vi "Auto Scroll Tree.vi"(8 "error in":errorcluster, 10 "TreeControl in":refnum<vi>, 11 "Recent Root Tags Map":refnum<vi>) -> (0 "error out":errorcluster)   [LabVIEW 2025, in "CAN-LIN Raw Bus Capture UI.lvlib"]
doc: "This VI creates a buffer, and checks if the buffer size is more then 19, then it deletes the oldest element, adds the new one to the end, and sets the TREE's top left cell to the oldest one. So the latest 20 element will be shown in the tree."
uses:
  CAN-LIN Raw Bus Capture UI.lvlib
  <vilib>/Utility/miscctls.llb/LVNodeAndColumnTypeDef.ctl
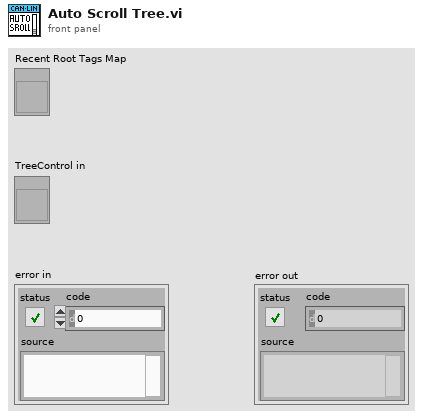
[diagram p1: front panel]
types:
  T1 = typedef "LVNodeAndColumnTypeDef.ctl" = cluster{"Node":string, "Column":i32}
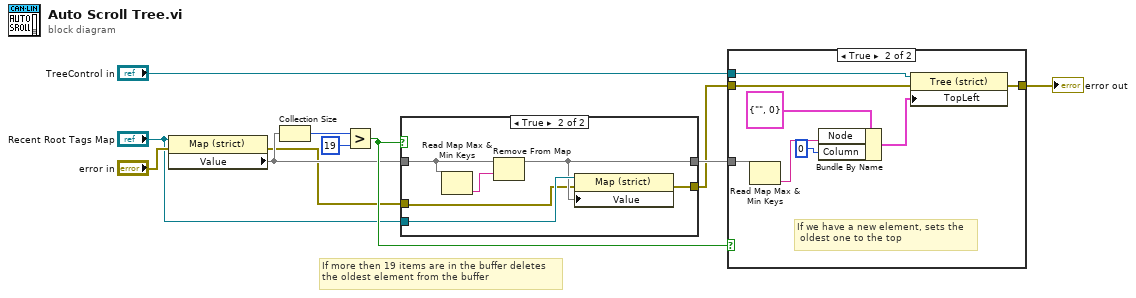
[diagram p0: block diagram]
diagram:
  # "If more then 19 items are in the buffer deletes\nthe oldest element from the buffer"
  n1 = property class="Map (strict)"(reference="Recent Root Tags Map", error in="error in") -> (error out=w2:errorcluster, "Value"=w6:map{string, string})  [unwired: 1 out]
  n2 = Collection Size(1:w6) -> (0:w7:i32)
  n3 = Greater?(x=w7, y=19) -> (0:w9:bool)
  n4 = case shown="True" w9 {
    tunnel: w6 -> [w13 w19]
    tunnel: [w13 w16] -> w5
    tunnel: "Recent Root Tags Map" -> [_ w17]
    tunnel: w2 -> [w12 w15]
    tunnel: [w12 w14] -> w1
    frame False {
    }
    frame True {
      n5 = Read Map Max & Min Keys(11:w19) -> (1:w18:string)  [unwired: 1 out]
      n6 = Remove From Map(10:w18, 11:w19) -> (3:w16:map{string, string})  [unwired: 2 out]
      n7 = property class="Map (strict)"(reference=w17, error in=w15, "Value"=w16) -> (error out=w14:errorcluster)  [unwired: 1 out]
    }
  }
  n8 = case shown="True" w9 {
    tunnel: [w20 w28] -> w11
    tunnel: "TreeControl in" -> [_ w27]
    tunnel: w1 -> [w20 w26]
    tunnel: w5 -> [_ w22]
    frame False {
    }
    frame True {
      # "If we have a new element, sets the\n oldest one to the top"
      n9 = Read Map Max & Min Keys(11:w22) -> (1:w21:string)  [unwired: 1 out]
      n10 = Bundle By Name(cluster=T1 {"Node"="", "Column"=0} ("Top Left Visible Cell"), "Node"=w21, "Column"=0) -> (w23:T1)
      n11 = property class="Tree (strict)"(reference=w27, error in=w26, "TopLeft"=w23) -> (error out=w28:errorcluster)  [unwired: 1 out]
    }
  }
  "error out" <- w11
